vi "LEUI_Create_Blink_Expected_LEDs.vi"(7 "Boolean":bool) -> (8 "Expect LED's Out":T2)   [LabVIEW 2016, in "Centauro.lvlib"]
uses:
  Projects/Centauro.lvlib
  type defs/LED Status OOB.ctl
  Functional Globals/Type Defs/State Action.ctl
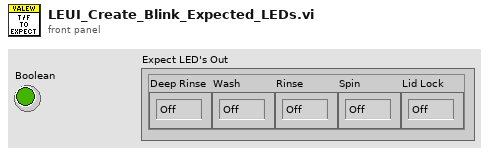
[diagram p1: front panel]
types:
  T1 = typedef "LED Status OOB.ctl" = enum32{"Off", "On", "Blink"}
  T2 = cluster{"Deep Rinse":T1, "Wash":T1, "Rinse":T1, "Spin":T1, "Lid Lock":T1}
  T3 = typedef "State Action.ctl" = enum16{"Get", "Set"}
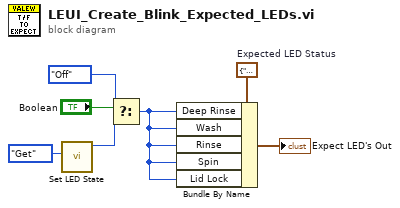
[diagram p0: block diagram]
diagram:
  w7 = T2 {"Deep Rinse"=enum."Off", "Wash"=enum."Off", "Rinse"=enum."Off", "Spin"=enum."Off", "Lid Lock"=enum."Off"}  # Expected LED Status
  n1 = call "Set LED State.vi"("Get/Set"=State_Action."Get") -> ("LED State Out"=w2:T1)  [unwired: 9 in, 1 out]
  n2 = Select(t=LED_Status_OOB."Off" ("Deep Rinse"), s="Boolean", f=w2) -> (s? t:f=w5:T1)
  n3 = Bundle By Name(cluster=w7, "Deep Rinse"=w5, "Wash"=w5, "Rinse"=w5, "Spin"=w5, "Lid Lock"=w5) -> (→"Expect LED's Out":T2)
